vi "CRYSet Optional Modules Front Panel.vi"(11 "Vi Ref In":refnum<vi> caption="Vi Ref") -> (3 "Vi Ref Out":refnum<vi> caption="Vi Ref")   [LabVIEW 2013]
doc: "Config File Reading/Writting\n\nPath \n ini File path\nRWFlag\n 0: no action\n 1: read\n 2: write"
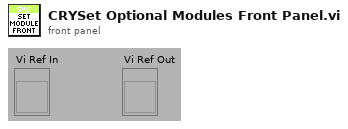
[diagram p1: front panel]
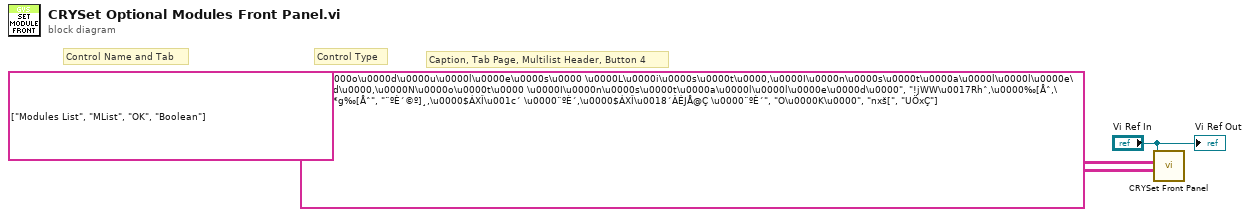
[diagram p0: block diagram]
diagram:
  # "Caption, Tab Page, Multilist Header, Button 4"
  # "Control Type"
  # "Control Name and Tab"
  n1 = call "CRYSet Front Panel.vi"("Caption(Boolean Text)"=string[][] [["M\u0000o\u0000d\u0000u\u0000l\u0000e\u0000s\u0000 \u0000L\u0000i\u0000s\u0000t\u0000,\u0000I\u0000n\u0000s\u0000t\u0000a\u0000l\u0000l\u0000e\u0000d\u0000,\u0000N\u0000o\u0000t\u0000 \u0000I\u0000n\u0000s\u0000t\u0000a\u0000l\u0000l\u0000e\u0000d\u0000", "!jWW\u0017Rhˆ,\u0000‰[Åˆ,\u0000*g‰[Åˆ", "¨ºÈ´©º]¸,\u0000$ÁXÎ\u001c´ \u0000¨ºÈ´,\u0000$ÁXÎ\u0018´ÀÉJÅ@Ç \u0000¨ºÈ´"], ["O\u0000K\u0000", "nxš[", "UÖxÇ"]], "Control ID and Type(Label Name, Type)"=string[][] [["Modules List", "MList"], ["OK", "Boolean"]], "Vi Ref"="Vi Ref In") -> ()  [unwired: 9 in]
  "Vi Ref Out" <- "Vi Ref In"
